vi "Create.vi"(8 "error in (no error)":errorcluster) -> (0 "error out":errorcluster, 3 "Controller out":refnum<class "Controller.lvclass">)   [LabVIEW 2020, in "UIHome.lvlib" / "Controller.lvclass"]
uses:
  Controller.lvclass
  Controller.lvclass/Controller.ctl
  View/View.lvclass
  C:/Users/N Tan/Documents/2-Prototypes/MVC/UIHome/View/View.lvclass
  C:/Users/N Tan/Documents/2-Prototypes/MVC/UIHome/iView/iView.lvclass
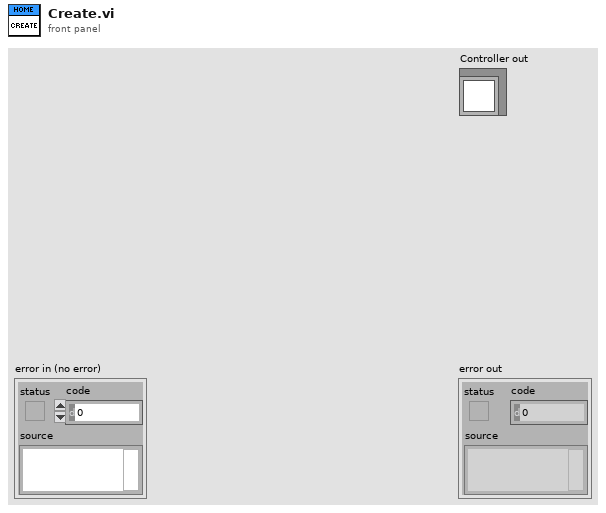
[diagram p1: front panel]
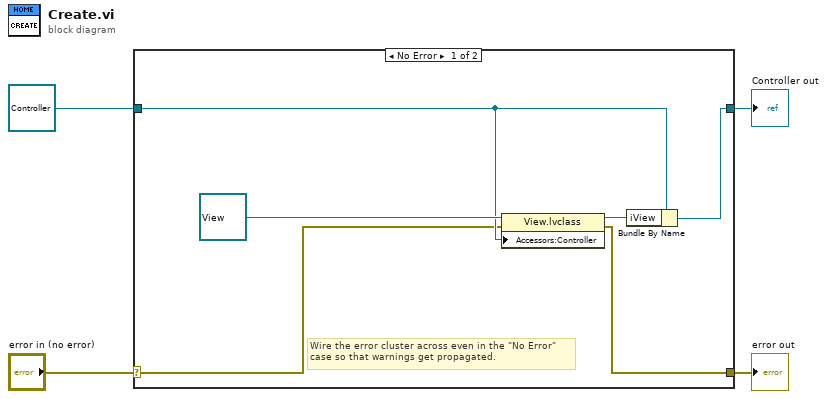
[diagram p0: block diagram]
diagram:
  n1 = case shown="No Error" "error in (no error)" {
    selector: "error in (no error)" -> [w6 w12]
    tunnel: [w5 w12] -> w3
    tunnel: [w7 w11] -> w2
    tunnel: refnum<class "Controller.lvclass"> refnum ("Controller in") -> [w8 w11]
    frame No Error {
      # "Wire the error cluster across even in the \"No Error\"\ncase so that warnings get propagated."
      n2 = property class="View.lvclass"(reference=refnum<class "View.lvclass"> refnum ("UIHome.lvlib:View.lvclass"), error in=w6, "Accessors:Controller"=w8) -> (reference out=w10:refnum<class "View.lvclass">, error out=w5:errorcluster)
      n3 = Bundle By Name(cluster=w8, "iView"=w10) -> (w7:refnum<class "Controller.lvclass">)
    }
    frame Error {
    }
  }
  "error out" <- w3
  "Controller out" <- w2
